vi "save.vi"(9 "Circles (Shape Detection 1)":T1(array[cluster]), 10 "Channel Names":string[](array[string])=["Channel 1", "Channel 2", "Channel 3", "Channel 4", "Channel 5"], 11 "File Name":path=path "C:/Documents and Settings/husmith/Desktop/CSVdata.csv") -> ()   [LabVIEW 2015]
uses:
  <vilib>/Utility/file.llb/Write To Spreadsheet File (DBL).vi
  <vilib>/Utility/file.llb/Write To Spreadsheet File (string).vi
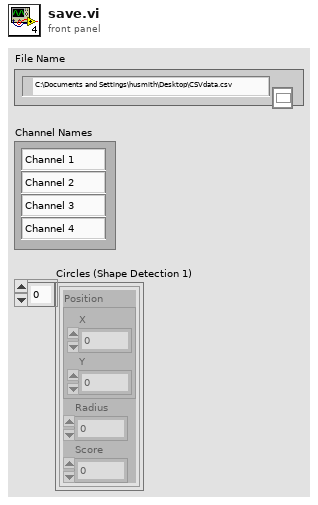
[diagram p1: front panel]
types:
  T1 = cluster{"Position":cluster{"X":sgl, "Y":sgl}, "Radius":dbl, "Score":dbl}[]
  T2 = cluster{"Position":cluster{"X":sgl, "Y":sgl}, "Radius":dbl, "Score":dbl}
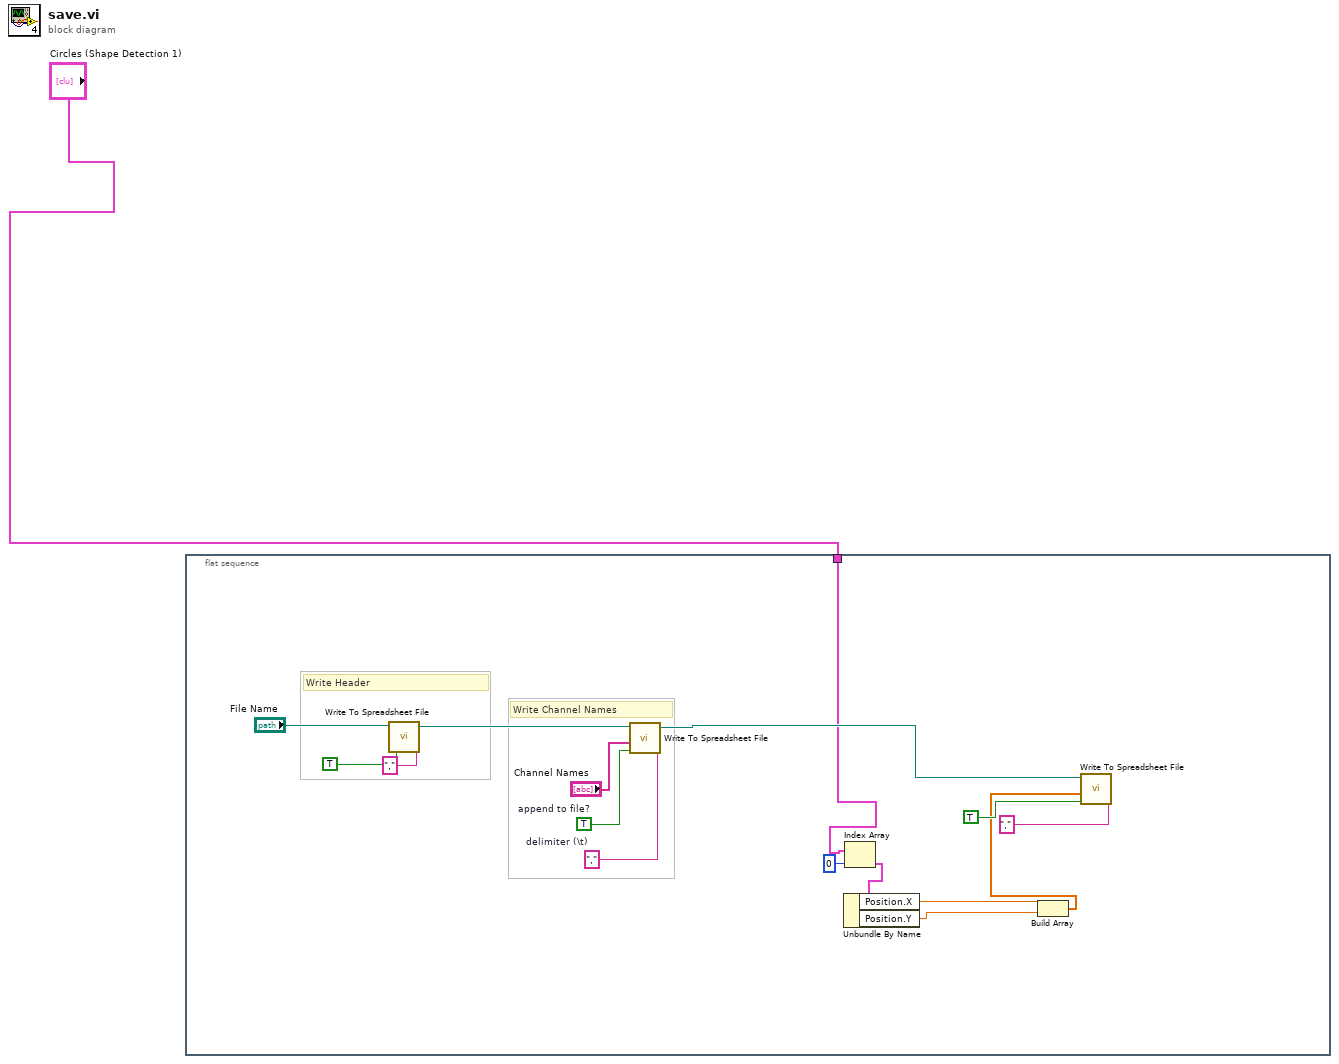
[diagram p0: block diagram]
diagram:
  n1 = flat-sequence {
    tunnel: "Circles (Shape Detection 1)" -> [w3]
    frame #0 {
      w13 = TRUE  # append to file?
      w14 = ","  # delimiter (\t)
      # "Write Header"
      # "Write Channel Names"
      n2 = call-poly <vilib>:"Write To Spreadsheet File.vi"("delimiter (\\t)"="," ("delimiter (\\t)"), "append to file? (new file:F)"=TRUE, "file path (dialog if empty)"="File Name") -> ("new file path (Not A Path if cancelled)"=w15:path)  [unwired: 4 in, 1 out]
      n3 = call-poly <vilib>:"Write To Spreadsheet File.vi"("delimiter (\\t)"=w14, "append to file? (new file:F)"=w13, "1D data"="Channel Names", "file path (dialog if empty)"=w15) -> ("new file path (Not A Path if cancelled)"=w17:path)  [unwired: 3 in, 1 out]
      n4 = Index Array(array=w3, index=0) -> (element=w8:T2)
      n5 = Unbundle By Name(w8) -> ("Position.X"=w6:sgl, "Position.Y"=w5:sgl)
      n6 = Build Array(w6, w5) -> (w4:sgl[])
      n7 = call-poly <vilib>:"Write To Spreadsheet File.vi"("delimiter (\\t)"="," ("delimiter (\\t)"), "append to file? (new file:F)"=TRUE, "1D data"=w4, "file path (dialog if empty)"=w17) -> ()  [unwired: 3 in, 2 out]
    }
  }
